vi "Execute.vi"(8 "error in (no error)":errorcluster, 10 "Motor in":refnum<class "Motor.lvclass">, 11 "Move in":refnum<class "Move-Relative.lvclass">) -> (0 "error out":errorcluster, 1 "Status message":string, 2 "Motor out":refnum<class "Motor.lvclass">, 3 "Move out":refnum<class "Move-Relative.lvclass">)   [LabVIEW 2013, in "PowderDeposition.lvlib" / "Move-Relative.lvclass"]
uses:
  Move-Relative.lvclass
  Motor/Motor.lvclass
  Move-Relative.lvclass/Move-Relative.ctl
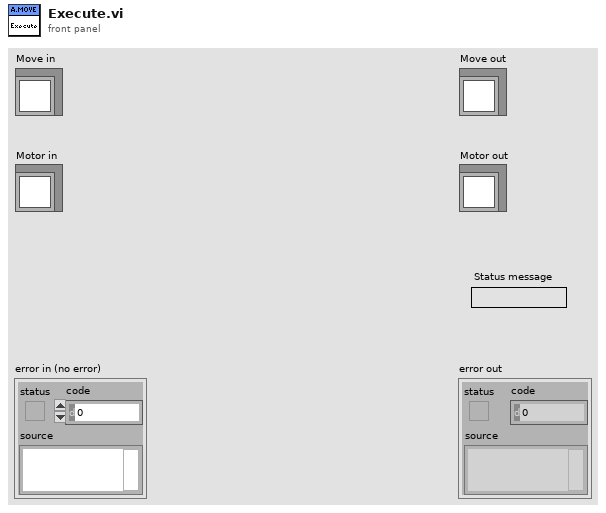
[diagram p1: front panel]
types:
  T1 = typedef "PowderDeposition.lvlib/Motor.lvclass/Units.ctl" = enum16{"-", "mm", "µm", "tr", "V"}
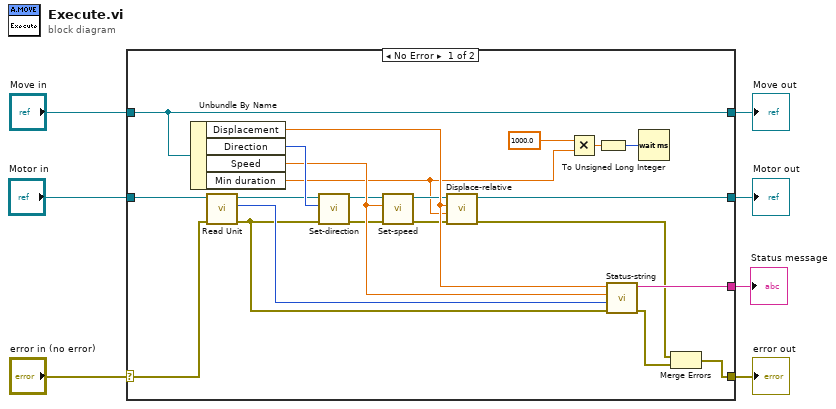
[diagram p0: block diagram]
diagram:
  n1 = case shown="No Error" "error in (no error)" {
    selector: "error in (no error)" -> [w22 w32]
    tunnel: [w20 w32] -> w6
    tunnel: [w29 w31] -> w4
    tunnel: "Move in" -> [w29 w31]
    tunnel: [w21 _] -> w3
    tunnel: "Motor in" -> [w23 w30]
    tunnel: [w28 w30] -> w1
    frame No Error {
      n2 = Unbundle By Name(w29) -> ("Displacement"=w15:dbl, "Direction"=w27:enum16{"Clockwise", "Counter-clockwise"}, "Speed"=w16:dbl, "Min duration"=w8:dbl)
      n3 = call-dynamic "Read Unit.vi"("error in (no error)"=w22, "Motor in"=w23) -> ("error out"=w9:errorcluster, "Unit"=w17:T1, "Motor out"=w14:refnum<class "Motor.lvclass">)  [unwired: 7 in]
      n4 = call-dynamic "Set-direction.vi"("error in (no error)"=w9, "Direction"=w27, "Motor in"=w14) -> ("error out"=w10:errorcluster, "Motor out"=w13:refnum<class "Motor.lvclass">)  [unwired: 7 in]
      n5 = call-dynamic "Set-speed.vi"("error in (no error)"=w10, "Speed"=w16, "Motor in"=w13) -> ("error out"=w11:errorcluster, "Motor out"=w12:refnum<class "Motor.lvclass">)  [unwired: 7 in]
      n6 = call-dynamic "Displace-relative.vi"("error in (no error)"=w11, "Min druation"=w8, "Displacement"=w15, "Motor in"=w12) -> ("error out"=w19:errorcluster, "Motor out"=w28:refnum<class "Motor.lvclass">)  [unwired: 6 in]
      n7 = Multiply(x=1000.0, y=w8) -> (x*y=w25:dbl)
      n8 = To Unsigned Long Integer(number=w25) -> (unsigned 32bit integer=w24:u32)
      n9 = call "Status-string.vi"("error in (no error)"=w9, "Unit"=w17, "Speed"=w16, "Displacement"=w15) -> ("error out"=w18:errorcluster, "Status string"=w21:string)  [unwired: 6 in]
      n10 = Wait (ms)(milliseconds to wait=w24) -> ()  [unwired: 1 out]
      n11 = Merge Errors(w19, w18) -> (w20:errorcluster)
    }
    frame Error {
    }
  }
  "error out" <- w6
  "Move out" <- w4
  "Status message" <- w3
  "Motor out" <- w1
